vi "Read Model.vi"(8 "error in (no error)":errorcluster, 11 "GEN40-38-LAN in":refnum<class "GEN40-38-LAN.lvclass">) -> (0 "error out":errorcluster, 2 "Model":string, 3 "GEN40-38-LAN out":refnum<class "GEN40-38-LAN.lvclass">)   [LabVIEW 2018, in "GEN40-38-LAN.lvlib" / "GEN40-38-LAN.lvclass"]
uses:
  GEN40-38-LAN.lvclass
  GEN40-38-LAN.lvclass/GEN40-38-LAN.ctl
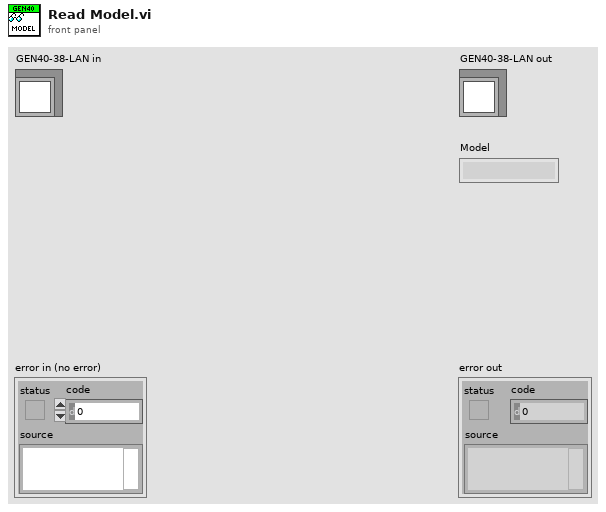
[diagram p1: front panel]
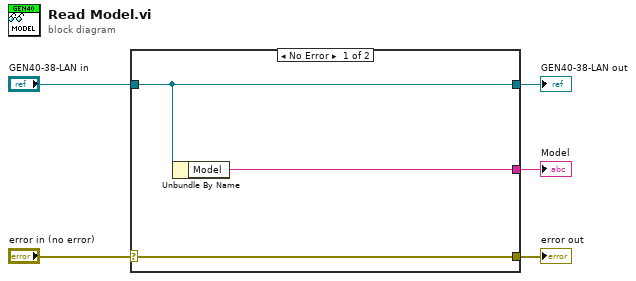
[diagram p0: block diagram]
diagram:
  n1 = case shown="No Error" "error in (no error)" {
    selector: "error in (no error)" -> [w8 w9]
    tunnel: [w8 w9] -> w4
    tunnel: [w7 w10] -> w2
    tunnel: "GEN40-38-LAN in" -> [w7 w10]
    tunnel: [w6 _] -> w1
    frame No Error {
      n2 = Unbundle By Name(w7) -> ("Model"=w6:string)
    }
    frame Error {
    }
  }
  "error out" <- w4
  "GEN40-38-LAN out" <- w2
  "Model" <- w1
